vi "Weather Simulator.vi"(11 "entrée d'erreur (pas d'erreur)":errorcluster) -> (6 "Graphe":dynamicdata(graph), 15 "sortie d'erreur":errorcluster)   [LabVIEW 2009]
doc: "Ce VI a généré une mesure de température et une mesure de tension sur un signal sinusoïdal à 50 kHz pour 5000 points. Ce VI sert de simulation dans le projet Station météo si aucun matériel n'est disponible."
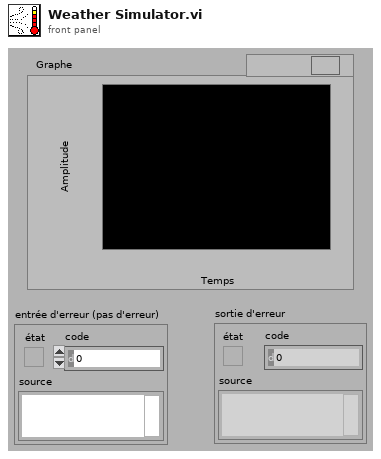
[diagram p1: front panel]
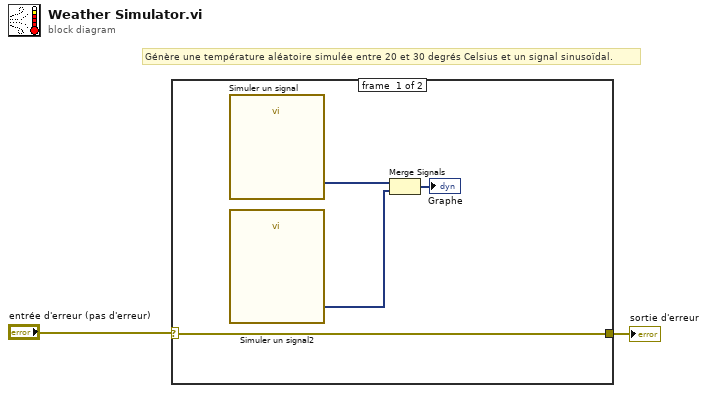
[diagram p0: block diagram]
diagram:
  # "Génère une température aléatoire simulée entre 20 et 30 degrés Celsius et un signal sinusoïdal."
  n1 = case "Structure Condition" shown="Pas d'erreur" "entrée d'erreur (pas d'erreur)" {
    selector: "entrée d'erreur (pas d'erreur)" -> [w6 w7]
    tunnel: [w6 w7] -> w1
    frame #0 {
      n2 = call "Simuler un signal"() -> ("Température"=w4:dynamicdata)  [unwired: 14 in, 1 out]
      n3 = call "Simuler un signal2"() -> ("Sinus"=w3:dynamicdata)  [unwired: 14 in, 1 out]
      n4 = Merge Signals ("Assembler des signaux")(w4, w3) -> (→"Graphe":dynamicdata)
    }
    frame #1 {
    }
  }
  "sortie d'erreur" <- w1
